vi "QDMH State to Queue Element.vi"(10 "State":string) -> (2 "QDSM Element":cluster{"State":string, "Variant Data":variant})   [LabVIEW 2009]
doc: "This VI has been replace by the polymorphic enqueue for the QDSM. However, it does illustrate a unique type of icon that could be used when a VI only has one input and one output.\n\nAAL 9/09"
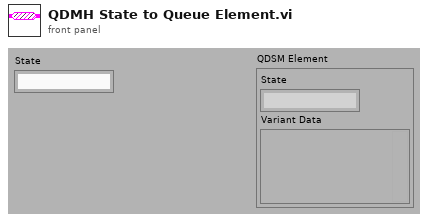
[diagram p1: front panel]
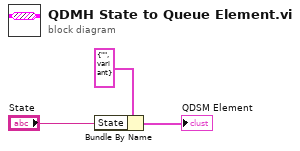
[diagram p0: block diagram]
diagram:
  n1 = Bundle By Name(cluster=cluster{"State":string, "Variant Data":variant} {"State"="", "Variant Data"=variant} ("QDSM Element"), "State"="State") -> (→"QDSM Element":cluster{"State":string, "Variant Data":variant})
